vi "Estimate Digit.vi"(4 "Denom Info":cluster{"Denom":i32, "Offset":i32}, 5 "A":T1) -> (0 "Estimated Digit":i32)   [LabVIEW 2025]
uses:
  Number.ctl
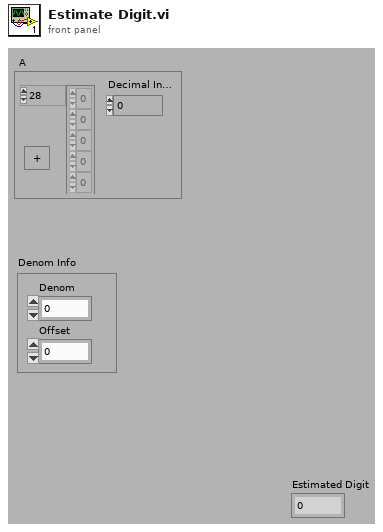
[diagram p1: front panel]
types:
  T1 = typedef "Number.ctl" = cluster{"Array Num":i8[], "Decimal Index":i32, "stop":bool}
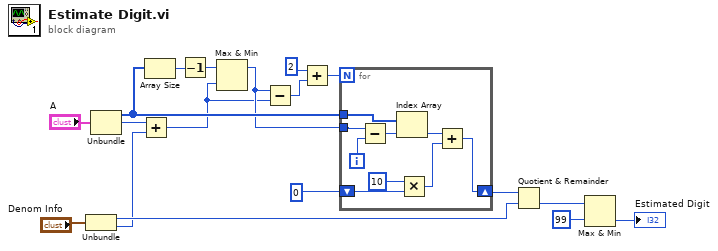
[diagram p0: block diagram]
diagram:
  n1 = Unbundle("Denom Info") -> ("Denom"=w2:i32, "Offset"=w1:i32)
  n2 = Unbundle("A") -> ("Array Num"=w13:i8[], "Decimal Index"=w15:i32)  [unwired: 1 out]
  n3 = Add(x=w15, y=w1) -> (x+y=w10:i32)
  n4 = Array Size(array=w13) -> (size(s)=w14:i32)
  n5 = Decrement(x=w14) -> (x-1=w12:i32)
  n6 = Max & Min(x=w12, y=w10) -> (max(x,y)=w11:i32)  [unwired: 1 out]
  n7 = Subtract(x=w11, y=w10) -> (x-y=w9:i32)
  n8 = Add(x=2 ("f"), y=w9) -> (x+y=w7:i32)
  n9 = for {
    N: w7 -> [_]
    tunnel: w11 -> [w27]
    tunnel: w13 -> [w24]
    shift-right: [w19] -> w16
    shift-left: 0 ("f") -> [w21]
    i -> [w26]
    n10 = Subtract(x=w27, y=w26) -> (x-y=w25:i32)
    n11 = Index Array(array=w24, index=w25) -> (element=w23:i8)
    n12 = Multiply(x=10, y=w21) -> (x*y=w22:i32)
    n13 = Add(x=w23, y=w22) -> (x+y=w19:i32)
  }
  n14 = Quotient & Remainder(x=w16, y=w2) -> (floor(x/y)=w6:i32)  [unwired: 1 out]
  n15 = Max & Min(x=w6, y=99) -> (min(x,y)=→"Estimated Digit":i32)  [unwired: 1 out]
